vi "RF voltage at 0 db atten. (FGV).vi"(8 "error in (no error)":errorcluster, 10 "Enum":enum16{"Read", "Write"}(ring), 11 "RF voltage at 0 dB atten.":dbl) -> (0 "error out":errorcluster, 3 "RF voltage at 0 dB atten.":dbl)   [LabVIEW 2014]
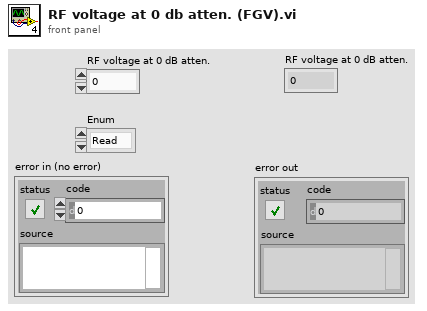
[diagram p1: front panel]
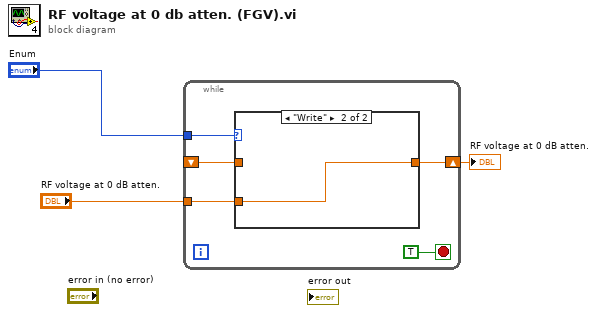
[diagram p0: block diagram]
diagram:
  n1 = while {
    tunnel: "Enum" -> [w8]
    tunnel: "RF voltage at 0 dB atten." -> [w6]
    shift-right: [w5] -> w1
    shift-left: _ -> [w4]
    stop <- TRUE stop-if-true
    n2 = case shown="\"Write\"" w8 {
      tunnel: w6 -> [_ w10]
      tunnel: [w9 w10] -> w5
      tunnel: w4 -> [w9 _]
      frame "Read", Default {
      }
      frame "Write" {
      }
    }
  }
  "RF voltage at 0 dB atten." <- w1
